vi "Vision Launcher.vi"() -> ()   [LabVIEW 2022 SP3]
uses:
  UDP Input.ctl
  Vision/Vision/Vision.lvclass
  C:/Program Files (x86)/National Instruments/LabVIEW 2022/vi.lib/ActorFramework/Actor/Actor.lvclass
  UDP Data Receiver/UDP Data Receiver Messages/Start Receiving Msg/Start Receiving Msg.lvclass/Start Receiving Msg.ctl
  <vilib>/ActorFramework/Message Enqueuer/Message Enqueuer.lvclass/Message Enqueuer.ctl
  <vilib>/ActorFramework/Message Enqueuer/Enqueue.vi
  UDP Data Receiver/UDP Data Receiver Messages/Start Receiving Msg/Start Receiving Msg.lvclass
  C:/Program Files (x86)/National Instruments/LabVIEW 2022/vi.lib/ActorFramework/Message/Message.lvclass
  UDP Data Receiver/UDP Data Receiver Messages/Stop Receiving Msg/Stop Receiving Msg.lvclass
  <vilib>/ActorFramework/Stop Msg/Stop Msg.lvclass
  <vilib>/ActorFramework/Message Priority Queue/Priority Enqueue.vi
  <vilib>/ActorFramework/Actor/Actor.lvclass
panel:
  in  "Stop":bool
  in  "Stop vision":bool
  in  "Send Request":bool
  in  "Input":T1={"Local IP"="", "Port"="10020", "Server IP"="224.5.23.2"}
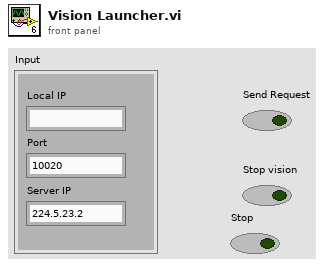
[diagram p1: front panel]
types:
  T1 = typedef "UDP Input.ctl" = cluster{"Local IP":string, "Port":string, "Server IP":string}
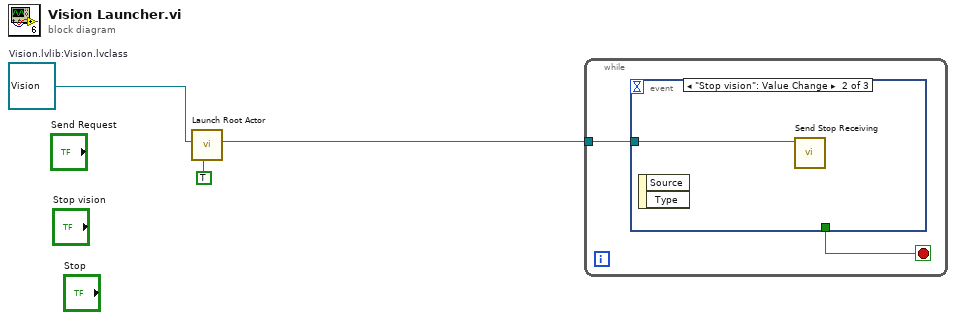
[diagram p0: block diagram]
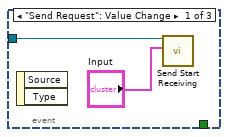
[diagram p2: hidden frame]
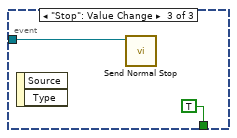
[diagram p3: hidden frame]
diagram:
  w1 = refnum<class "Vision.lvclass"> refnum  # Vision.lvlib:Vision.lvclass
  n1 = call <vilib>:"Launch Root Actor.vi"("Open Actor Core front panel? (F)"=TRUE, "Actor"=w1) -> ("Actor's Enqueuer"=w2:refnum<class "Message Enqueuer.lvclass">)  [unwired: 8 in, 1 out]
  n2 = while {
    tunnel: w2 -> [w5]
    stop <- w4 stop-if-true
    n3 = event shown="[1] \"Stop vision\": Value Change" {
      selector: _ -> [_ _ _]
      dyn-events: _ -> [_ _ _]
      timeout: _ -> [_ _ _]
      tunnel: w5 -> [w7 w8 w10]
      tunnel: [_ _ TRUE] -> w4
      event "Send Request": Value Change {
        n4 = event-data() -> ()  [unwired: 1 in, 2 out]
        n5 = call "Send Start Receiving.vi"("Input"="Input", "Message Enqueuer"=w7) -> ()  [unwired: 8 in, 2 out]
      }
      event "Stop vision": Value Change {
        n6 = event-data() -> ()  [unwired: 1 in, 2 out]
        n7 = call "Send Stop Receiving.vi"("Message Enqueuer"=w8) -> ()  [unwired: 9 in, 2 out]
      }
      event "Stop": Value Change {
        n8 = event-data() -> ()  [unwired: 1 in, 2 out]
        n9 = call <vilib>:"Send Normal Stop.vi"("Message Enqueuer"=w10) -> ()  [unwired: 10 in, 1 out]
      }
    }
  }
